vi "SeCrTs-RT_Sequence_Main.vi"(8 "error in":errorcluster, 11 "Message Queue":refnum<queue>) -> (0 "error out":errorcluster)   [LabVIEW 2022 SP3]
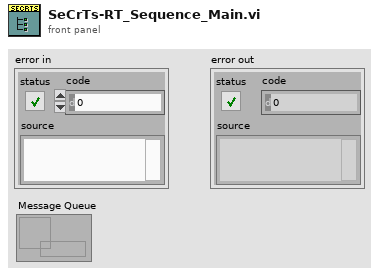
[diagram p1: front panel]
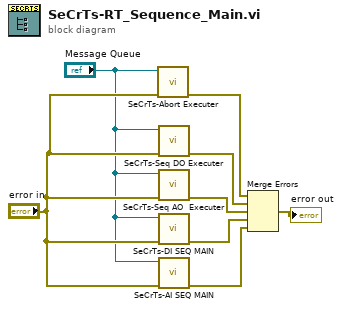
[diagram p0: block diagram]
diagram:
  n1 = call "SeCrTs-Abort Executer.vi"("error in"="error in", "Message Queue"="Message Queue") -> ("error IO"=w2:errorcluster)  [unwired: 9 in]
  n2 = call "SeCrTs-Seq DO Executer .vi"("error in"="error in", "Message Queue"="Message Queue") -> ("error IO"=w8:errorcluster)  [unwired: 9 in]
  n3 = call "SeCrTs-Seq AO  Executer.vi"("error in"="error in", "Message Queue"="Message Queue") -> ("error IO"=w7:errorcluster)  [unwired: 9 in]
  n4 = call "SeCrTs-DI SEQ MAIN.vi"("error in"="error in", "Message Queue"="Message Queue") -> ("error Out"=w6:errorcluster)  [unwired: 9 in]
  n5 = call "SeCrTs-AI SEQ MAIN.vi"("error IO"="error in", "Message Queue"="Message Queue") -> ("error Out"=w5:errorcluster)  [unwired: 9 in]
  n6 = Merge Errors(w2, w8, w7, w6, w5) -> (→"error out":errorcluster)
